vi "Read Wärmepumpe.Parameter.vi"(8 "error in (no error)":errorcluster, 11 "Wärmepumpe in":refnum<class "Wärmepumpe.lvclass">) -> (0 "error out":errorcluster, 2 "Wärmepumpe.Parameter":T1, 3 "Wärmepumpe out":refnum<class "Wärmepumpe.lvclass">)   [LabVIEW 2016, in "Wärmepumpe.lvclass"]
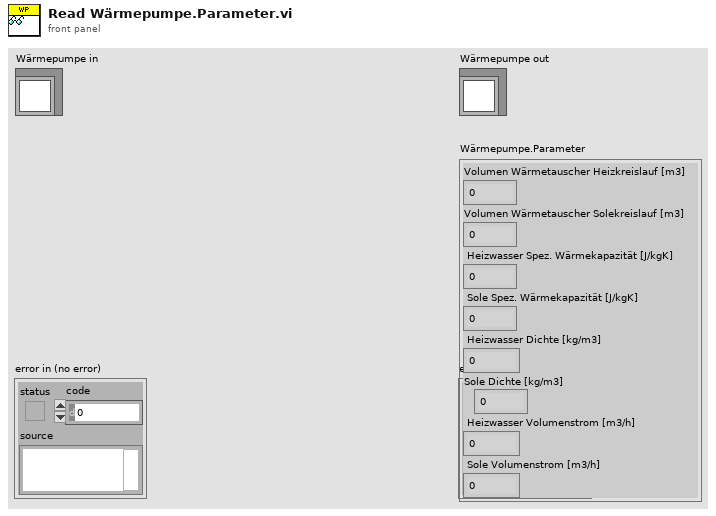
[diagram p1: front panel]
types:
  T1 = cluster{"Volumen Wärmetauscher Heizkreislauf [m3]":dbl, "Volumen Wärmetauscher Solekreislauf [m3]":dbl, " Heizwasser Spez. Wärmekapazität [J/kgK]":dbl, " Sole Spez. Wärmekapazität [J/kgK]":dbl, " Heizwasser Dichte [kg/m3]":dbl, "Sole Dichte [kg/m3] ":dbl, " Heizwasser Volumenstrom [m3/h]":dbl, " Sole Volumenstrom [m3/h]":dbl}
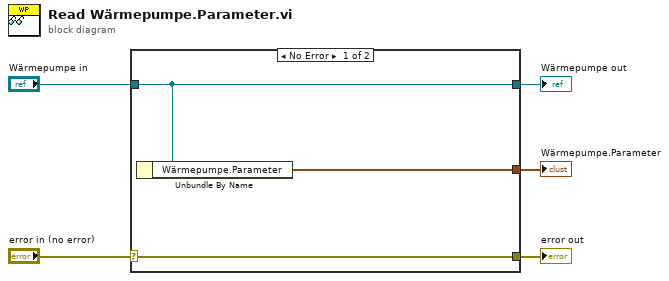
[diagram p0: block diagram]
diagram:
  n1 = case shown="No Error" "error in (no error)" {
    selector: "error in (no error)" -> [w8 w9]
    tunnel: [w8 w9] -> w4
    tunnel: [w7 w10] -> w2
    tunnel: "Wärmepumpe in" -> [w7 w10]
    tunnel: [w6 _] -> w1
    frame No Error {
      n2 = Unbundle By Name(w7) -> ("Wärmepumpe.Parameter"=w6:T1)
    }
    frame Error {
    }
  }
  "error out" <- w4
  "Wärmepumpe out" <- w2
  "Wärmepumpe.Parameter" <- w1
